vi "lowpass filtre.vi"(8 "in_k":dbl, 10 "TS":dbl, 11 "TF":dbl) -> (0 "Filtre output":dbl)   [LabVIEW 2021]
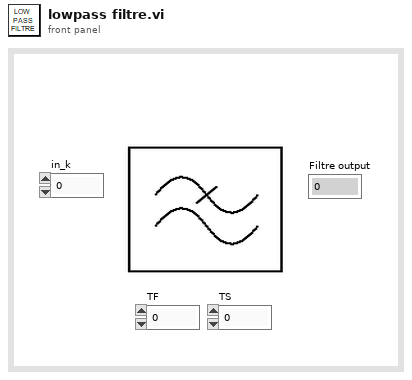
[diagram p1: front panel]
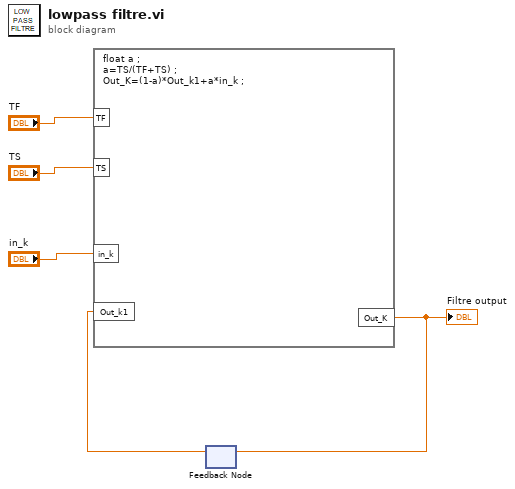
[diagram p0: block diagram]
diagram:
  n1 = feedback #1() -> (w2:dbl)  [unwired: 1 in]
  n2 = formula code="float a ;\na=TS/(TF+TS) ;\nOut_K=(1-a)*Out_k1+a*in_k ;"("TF"="TF", "TS"="TS", "in_k"="in_k", "Out_k1"=w2) -> ("Out_K"=w1:dbl)
  "Filtre output" <- w1
  n3 = feedback-in #1(w1) -> ()
